vi "Utility Parse Pressure Compensation.vi"(8 "error in (no error)":errorcluster, 11 "Input String":string) -> (0 "error out":errorcluster, 3 "Pressure Compensation (PSI)":i32)   [LabVIEW 2020, in "ChromTech Series I Drivers.lvlib"]
uses:
  <instrlib>/RxnRover/ChromtechSeriesIDriver/ChromTech Series I Drivers.lvlib
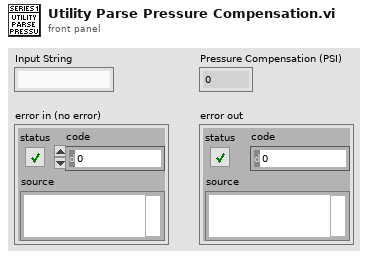
[diagram p1: front panel]
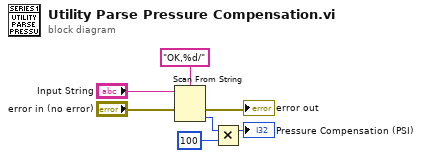
[diagram p0: block diagram]
diagram:
  n1 = Scan From String(format string="OK,%d/", input string="Input String", error in="error in (no error)") -> (error out=→"error out":errorcluster, output 1=w3:i32)  [unwired: 2 in, 2 out]
  n2 = Multiply(x=w3, y=100) -> (x*y=→"Pressure Compensation (PSI)":i32)
